vi "Is VI running.vi"(11 "VI name":string) -> (0 "error out":errorcluster, 3 "VI is running":bool)   [LabVIEW 2017]
doc: "SciScan 1.2 160622"
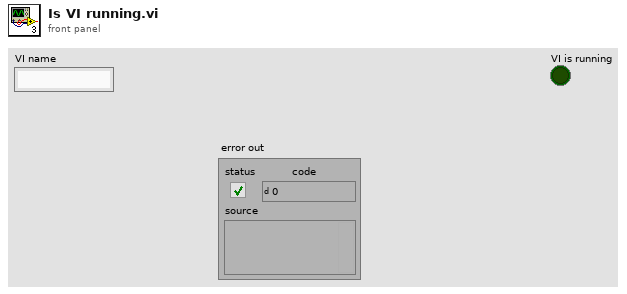
[diagram p1: front panel]
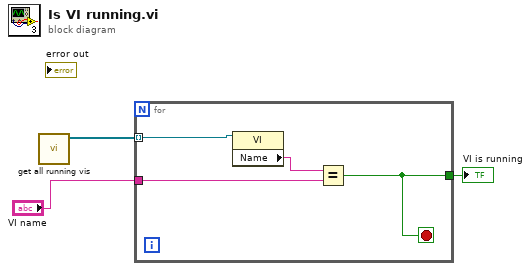
[diagram p0: block diagram]
diagram:
  n1 = call "get all running vis.vi"() -> ("RunningVIRefs"=w3:refnum<vi>[])  [unwired: 11 in]
  n2 = for {
    tunnel: w3 -> [w7] mode=indexing
    tunnel: "VI name" -> [w5]
    tunnel: [w4] -> w1
    stop <- w4 stop-if-true
    n3 = property class="VI"(reference=w7) -> ("Name"=w6:string)  [unwired: 1 in, 2 out]
    n4 = Equal?(x=w6, y=w5) -> (x = y?=w4:bool)
  }
  "VI is running" <- w1
